vi "get_number_of_channels.vi"(8 "error in (no error)":errorcluster, 11 "SignalReaderDL091205FPGA in":refnum<class "SignalReaderDL091205FPGA.lvclass">) -> (0 "error out":errorcluster, 2 "number of channels":i32, 3 "SignalReaderDL091205FPGA out":refnum<class "SignalReaderDL091205FPGA.lvclass">)   [LabVIEW 2010, in "SignalReaderDL091205FPGA.lvclass"]
uses:
  SignalReaderDL091205FPGA.lvclass
  SignalReaderDL091205FPGA.lvclass/SignalReaderDL091205FPGA.ctl
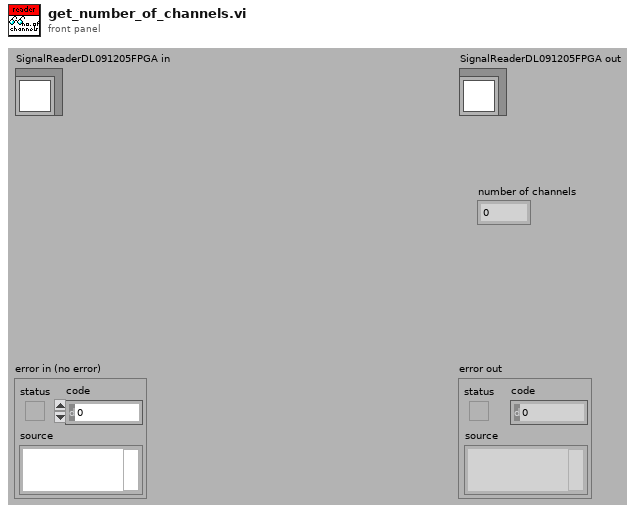
[diagram p1: front panel]
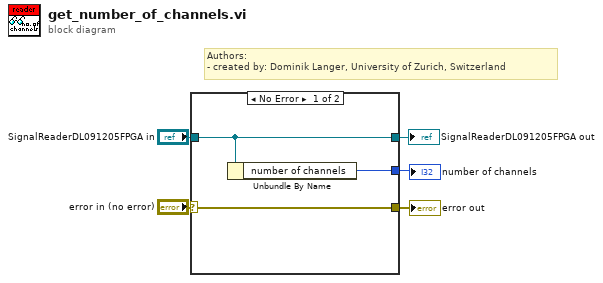
[diagram p0: block diagram]
diagram:
  # "Authors: \n- created by: Dominik Langer, University of Zurich, Switzerland"
  n1 = case shown="No Error" "error in (no error)" {
    selector: "error in (no error)" -> [w8 w10]
    tunnel: [w8 w10] -> w4
    tunnel: "SignalReaderDL091205FPGA in" -> [w7 w9]
    tunnel: [w7 w9] -> w2
    tunnel: [w6 _] -> w1
    frame No Error {
      n2 = Unbundle By Name(w7) -> ("number of channels"=w6:i32)
    }
    frame Error {
    }
  }
  "error out" <- w4
  "SignalReaderDL091205FPGA out" <- w2
  "number of channels" <- w1
